vi "results_interface.vi"() -> ()   [LabVIEW 2015]
panel:
  in  "Tab Control":enum32{"Controls", "Insigts", "Debug"}(tab)
  out "Cleaning Up":bool
  out "Calculating Sessions":bool
  out "Total Rate":string
  in  "Velocity Maximum":dbl=100.0 min=0.0 max=100.0
  in  "Experiment ID":string="All"
  in  "Lower Timestamp":timestamp=timestamp(3455817549.4224453 s since 1904-01-01)
  in  "Upper Timestamp":timestamp=timestamp(4308844760.779092 s since 1904-01-01)
  in  "Upper Integer Timestamp":i64=2225999960000 min=1340137854565 max=2040137854565 step=10000000
  in  "Lower Integer Timestamp":i64=1372972749000 min=1340137854565 max=2062085784667 step=10000000
  in  "Dust ID":string="Any"
  in  "Esstimate Dust Quality":cluster{i32, i32}(slide)={2, 5} scale=0.0..5.0
  out "Running":bool
  out "Finished Sessions":bool
  out "Valid Path":bool
  in  "Estimate Session Quality":cluster{i32, i32}(slide)={2, 5} scale=0.0..5.0
  in  "Dust Material":string(combo)="Any Material"
  in  "Velocity Minimun":dbl min=0.0 max=100.0
  in  "Path":path=path "C:/Users/17208/Dust-Accelerator-Database-Analysis/generate_sessions.py"
  in  "End Program":bool
  in  "Calculate Results":bool
  out "?":string="Session Quality Explanation"
  out "?":string="Vecloty Bins Explanation"
  in  "Calculate Results":bool
  in  "Tab Control 2":enum32{"Results Insights", "Results Breakdown"}(tab)
  in  "Tab Control 4":enum32{"Rates", "Particles", "Runtime"}(tab)
  out "results_rates.png":picture
  out "results_particle_count.png":picture
  out "results_runtime.png":picture
  in  "Tab Control 3":T1(tab)
  out "Session Quality Breakdown":picture
  out "Session Particle Quality Breakdown":picture
  out "Session Duration Breakdown":picture
  out "Session Dust Event Count Breakdown":picture
  out "Results Output":string
  out "Request":string
  out "Results Error/Debug":string
  out "Session Generator Output":string
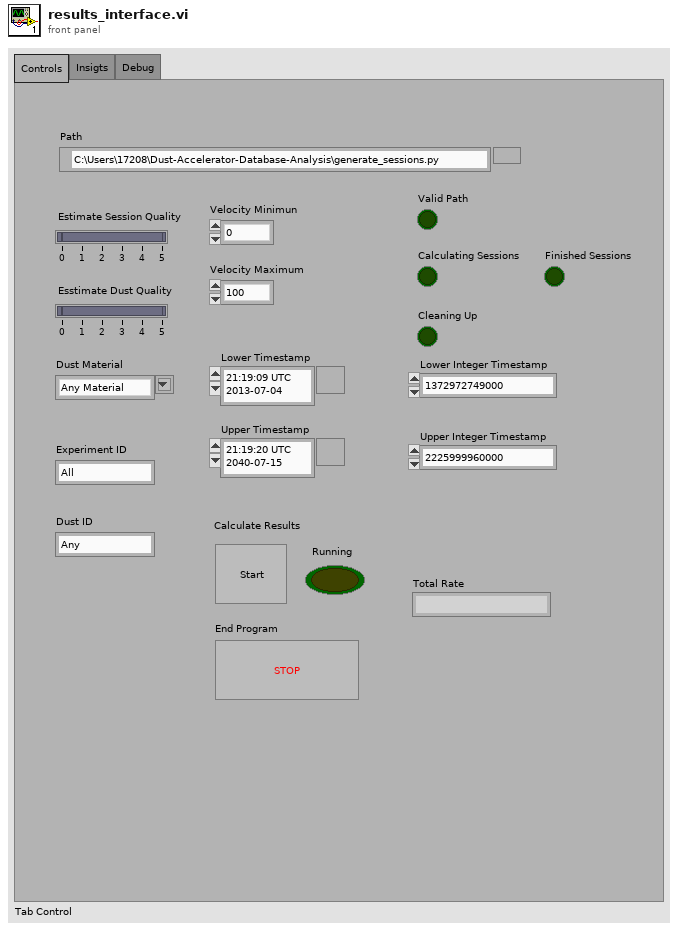
[diagram p1: front panel]
types:
  T1 = enum32{"Session Quality ", "Particle Quality", "Session Duration", "Session Event Counts"}
  T2 = cluster{string, string, string, string, string, string, string}
  T3 = cluster{"Velocity Minimun ":dbl, "Velocity Maximum":dbl}
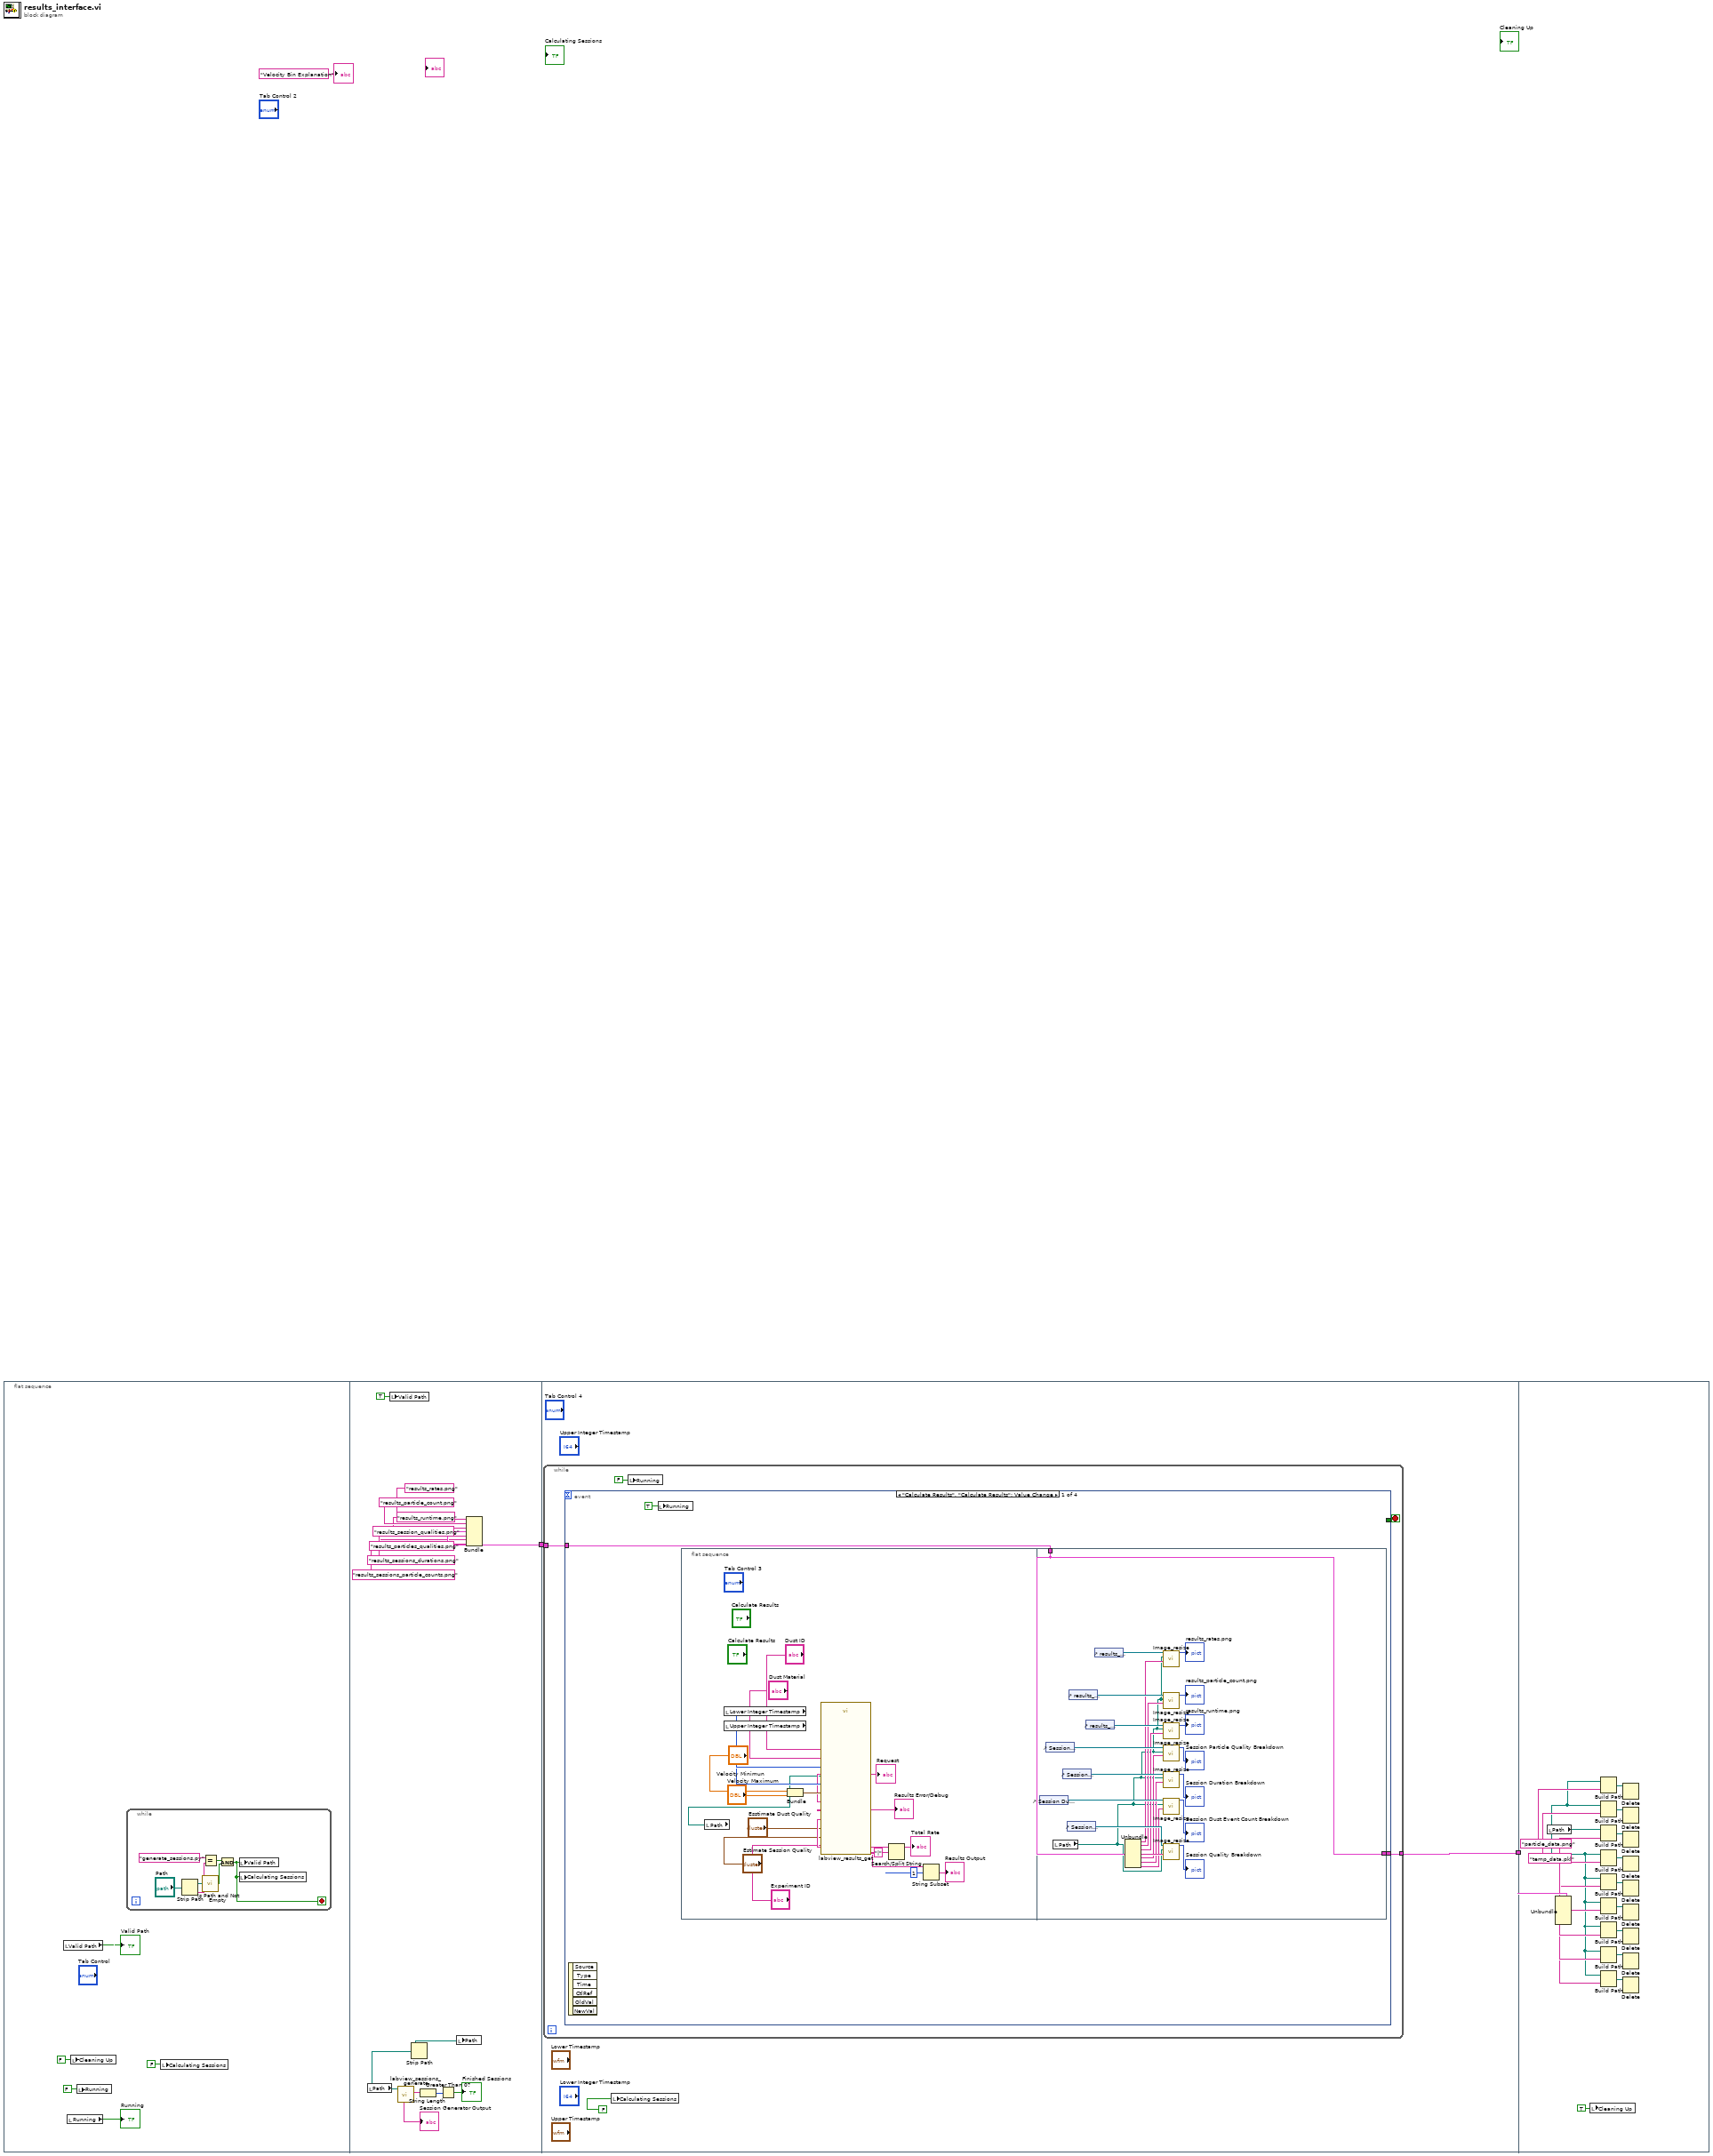
[diagram p0: block diagram]
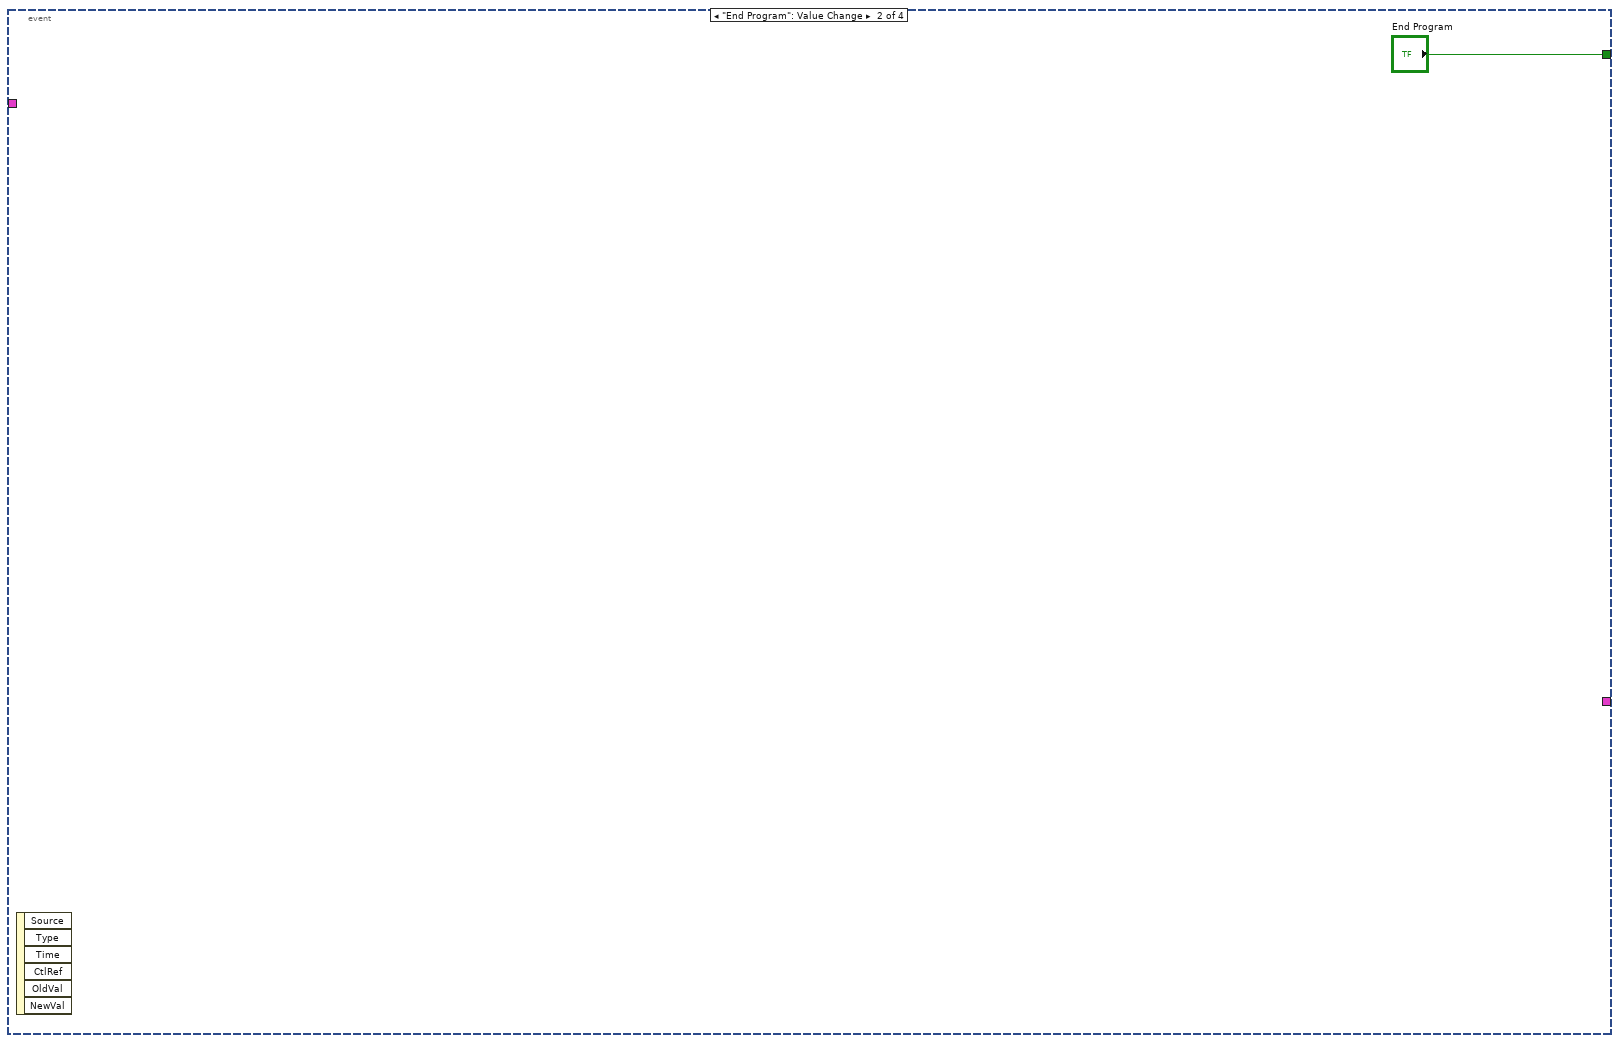
[diagram p2: hidden frame]
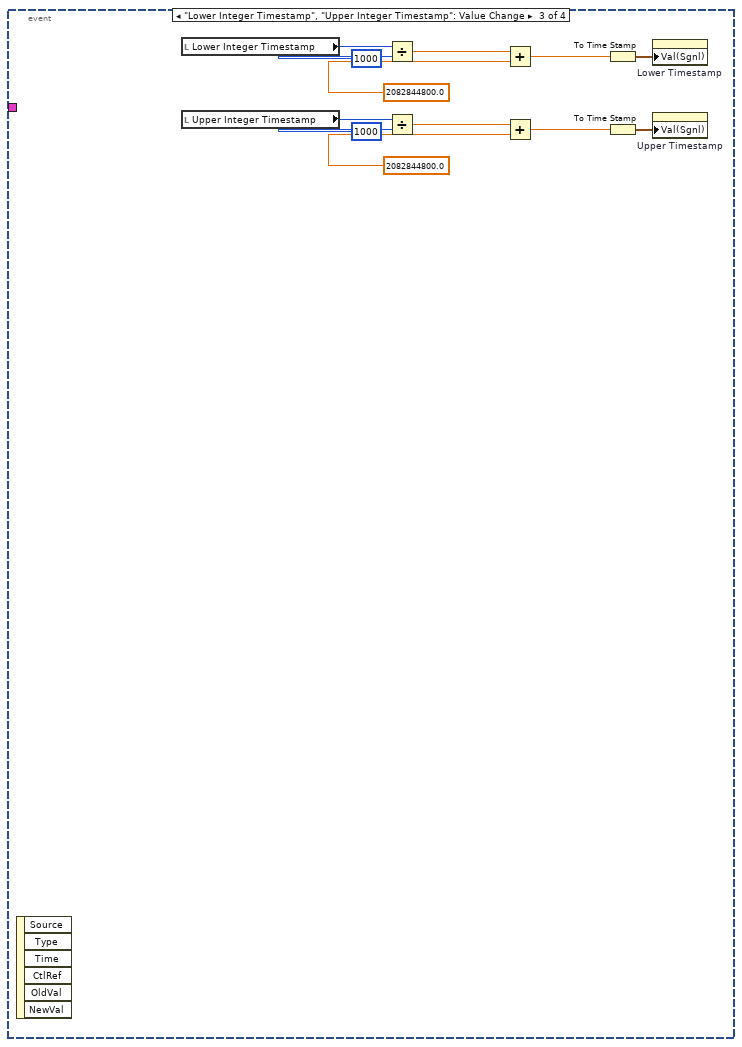
[diagram p3: hidden frame]
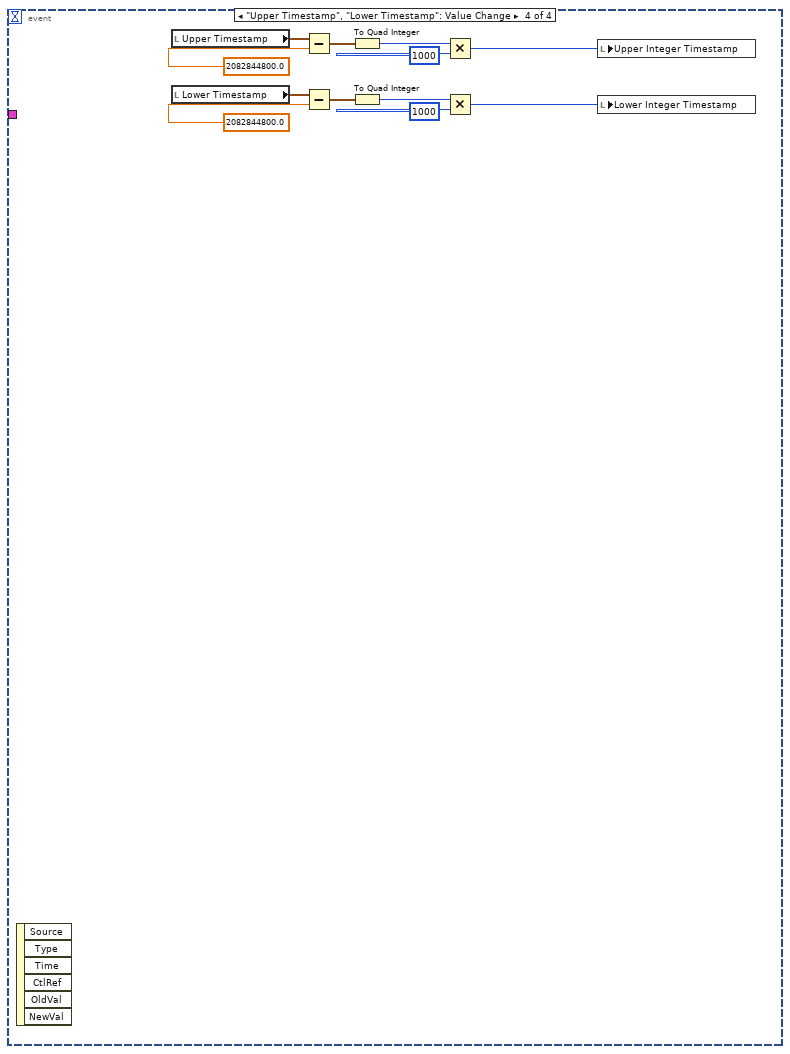
[diagram p4: hidden frame]
diagram:
  n1 = flat-sequence {
    tunnel: [w25] -> w2
    tunnel: w2 -> [w32]
    tunnel: [w31] -> w1
    tunnel: w1 -> [w116]
    frame #0 {
      n2 = local read "Valid Path"() -> (→"Valid Path":bool)
      n3 = local read "Running"() -> (→"Running":bool)
      n4 = local write "Cleaning Up"(FALSE ("Cleaning Up")) -> ()
      n5 = local write "Running"(FALSE) -> ()
      n6 = while {
        stop <- w9 stop-if-true
        n7 = Strip Path(path="Path") -> (stripped path=w10:path, name=w15:string)
        n8 = Equal?(x="generate_sessions.py", y=w15) -> (x = y?=w13:bool)
        n9 = call <vilib>:"Is Path and Not Empty.vi"("path"=w10) -> ("Is Path and Not Empty?"=w12:bool)  [unwired: 4 in]
        n10 = And(x=w13, y=w12) -> (x .and. y?=w9:bool)
        n11 = local write "Valid Path"(w9) -> ()
        n12 = local write "Calculating Sessions"(w9) -> ()
      }
      n13 = local write "Calculating Sessions"(FALSE ("Calculating Sessions")) -> ()
    }
    frame #1 {
      n14 = local read "Path"() -> (w17:path)
      n15 = local write "Valid Path"(TRUE) -> ()
      n16 = call "labview_sessions_generate.vi"("Path"=w17) -> ("Session Generator Output"=w29:string)  [unwired: 10 in]
      "Session Generator Output" <- w29
      n17 = Strip Path(path=w17) -> (stripped path=w16:path)  [unwired: 1 out]
      n18 = String Length(string=w29) -> (length=w28:i32)
      n19 = Greater Than 0?(x=w28) -> (x > 0?=→"Finished Sessions":bool)
      n20 = local write "Path"(w16) -> ()
      n21 = Bundle("results_rates.png", "results_particle_count.png", "results_runtime.png", "results_session_qualities.png", "results_particles_qualities.png", "results_sessions_durations.png", "results_sessions_particle_counts.png") -> (w25:T2)  [unwired: 1 in]
    }
    frame #2 {
      n22 = while {
        tunnel: w32 -> [w35]
        tunnel: [w34] -> w31
        stop <- w33 stop-if-true
        n23 = event shown="[0] \"Calculate Results\", \"Calculate Results\": Value Change" {
          selector: _ -> [_ _ _ _]
          dyn-events: _ -> [_ _ _ _]
          timeout: _ -> [_ _ _ _]
          tunnel: [_ "End Program" _ _] -> w33
          tunnel: w35 -> [w38 _ _ _]
          tunnel: [w37 _ _ _] -> w34
          event "Calculate Results", "Calculate Results": Value Change {
            n24 = event-data() -> ()  [unwired: 1 in, 6 out]
            n25 = local write "Running"(TRUE) -> ()
            n26 = flat-sequence {
              tunnel: w38 -> [w81]
              tunnel: [w81] -> w37
              frame #0 {
                n27 = local read "Path"() -> (w40:path)
                n28 = local read "Lower Integer Timestamp"() -> (w52:i64)
                n29 = local read "Upper Integer Timestamp"() -> (w51:i64)
                n30 = Bundle("Velocity Minimun"="Velocity Minimun", "Velocity Maximum"="Velocity Maximum") -> (w56:T3)  [unwired: 1 in]
                n31 = call "labview_results_get.vi"("Path"=w40, "Dust ID"="Dust ID", "Upper Timestamp"=w51, "Velocity Limits"=w56, "Lower Timestamp"=w52, "Particle Quality"="Esstimate Dust Quality", "Session Quality"="Estimate Session Quality", "Experiment ID"="Experiment ID", "Dust Material"="Dust Material") -> ("Results Output"=w57:string, "Results Error/Debug"=→"Results Error/Debug":string, "Request"=→"Request":string)  [unwired: 16 in]
                n32 = Search/Split String(string=w57, search string/char (-)="|") -> (substring before match=→"Total Rate":string, match + rest of string=w42:string)  [unwired: 1 in, 1 out]
                n33 = String Subset(string=w42, offset (0)=1) -> (substring=→"Results Output":string)  [unwired: 1 in]
              }
              frame #1 {
                n34 = control-ref of="Session Dust Event Count Breakdown"() -> (w67:refnum<vi>)
                n35 = control-ref of="Session Particle Quality Breakdown"() -> (w69:refnum<vi>)
                n36 = local read "Path"() -> (w59:path)
                n37 = control-ref of="Session Duration Breakdown"() -> (w68:refnum<vi>)
                n38 = control-ref of="Session Quality Breakdown"() -> (w70:refnum<vi>)
                n39 = control-ref of="results_particle_count.png"() -> (w72:refnum<vi>)
                n40 = control-ref of="results_runtime.png"() -> (w71:refnum<vi>)
                n41 = control-ref of="results_rates.png"() -> (w73:refnum<vi>)
                n42 = Unbundle(w81) -> (w66:string, w65:string, w64:string, w63:string, w62:string, w61:string, w60:string)
                n43 = call "Image_resize.vi"("String"=w66, "stripped path"=w59, "Picture in"=w73) -> ("2D Picture"=→"results_rates.png":picture)  [unwired: 8 in]
                n44 = call "Image_resize.vi"("String"=w65, "stripped path"=w59, "Picture in"=w72) -> ("2D Picture"=→"results_particle_count.png":picture)  [unwired: 8 in]
                n45 = call "Image_resize.vi"("String"=w64, "stripped path"=w59, "Picture in"=w71) -> ("2D Picture"=→"results_runtime.png":picture)  [unwired: 8 in]
                n46 = call "Image_resize.vi"("String"=w62, "stripped path"=w59, "Picture in"=w69) -> ("2D Picture"=→"Session Particle Quality Breakdown":picture)  [unwired: 8 in]
                n47 = call "Image_resize.vi"("String"=w61, "stripped path"=w59, "Picture in"=w68) -> ("2D Picture"=→"Session Duration Breakdown":picture)  [unwired: 8 in]
                n48 = call "Image_resize.vi"("String"=w60, "stripped path"=w59, "Picture in"=w67) -> ("2D Picture"=→"Session Dust Event Count Breakdown":picture)  [unwired: 8 in]
                n49 = call "Image_resize.vi"("String"=w63, "stripped path"=w59, "Picture in"=w70) -> ("2D Picture"=→"Session Quality Breakdown":picture)  [unwired: 8 in]
              }
            }
          }
          event "End Program": Value Change {
            n50 = event-data() -> ()  [unwired: 1 in, 6 out]
          }
          event "Lower Integer Timestamp", "Upper Integer Timestamp": Value Change {
            n51 = event-data() -> ()  [unwired: 1 in, 6 out]
            n52 = local read "Lower Integer Timestamp"() -> (w93:i64)
            n53 = local read "Upper Integer Timestamp"() -> (w91:i64)
            n54 = Divide(x=w93, y=1000) -> (x/y=w85:dbl)
            n55 = Divide(x=w91, y=1000) -> (x/y=w87:dbl)
            n56 = Add(x=w85, y=2082844800.0) -> (x+y=w83:dbl)
            n57 = Add(x=w87, y=2082844800.0) -> (x+y=w86:dbl)
            n58 = To Time Stamp(1:w83) -> (0:w89:timestamp)
            n59 = To Time Stamp(1:w86) -> (0:w90:timestamp)
            n60 = property on="Lower Timestamp" class="AbsTime (strict)"("Val(Sgnl)"=w89) -> ()  [unwired: 2 in, 2 out]
            n61 = property on="Upper Timestamp" class="AbsTime (strict)"("Val(Sgnl)"=w90) -> ()  [unwired: 2 in, 2 out]
          }
          event "Upper Timestamp", "Lower Timestamp": Value Change {
            n62 = event-data() -> ()  [unwired: 1 in, 6 out]
            n63 = local read "Upper Timestamp"() -> (w95:timestamp)
            n64 = local read "Lower Timestamp"() -> (w96:timestamp)
            n65 = Subtract(x=w95, y=2082844800.0) -> (x-y=w102:timestamp)
            n66 = Subtract(x=w96, y=2082844800.0) -> (x-y=w103:timestamp)
            n67 = To Quad Integer(1:w102) -> (0:w99:i64)
            n68 = To Quad Integer(1:w103) -> (0:w101:i64)
            n69 = Multiply(x=w99, y=1000) -> (x*y=w98:i64)
            n70 = Multiply(x=w101, y=1000) -> (x*y=w100:i64)
            n71 = local write "Upper Integer Timestamp"(w98) -> ()
            n72 = local write "Lower Integer Timestamp"(w100) -> ()
          }
        }
        n73 = local write "Running"(FALSE ("Boolean")) -> ()
      }
      n74 = local write "Calculating Sessions"(FALSE ("Calculating Sessions")) -> ()
    }
    frame #3 {
      n75 = local read "Path"() -> (w107:path)
      n76 = Unbundle(w116) -> (w115:string, w114:string, w113:string, w112:string, w111:string, w110:string, w109:string)
      n77 = local write "Cleaning Up"(TRUE ("Cleaning Up")) -> ()
      n78 = Build Path(base path=w107, name or relative path="particle_data.png") -> (appended path=w125:path)
      n79 = Build Path(base path=w107, name or relative path="temp_data.pkl") -> (appended path=w127:path)
      n80 = Build Path(base path=w107, name or relative path=w115) -> (appended path=w122:path)
      n81 = Build Path(base path=w107, name or relative path=w114) -> (appended path=w121:path)
      n82 = Build Path(base path=w107, name or relative path=w113) -> (appended path=w123:path)
      n83 = Build Path(base path=w107, name or relative path=w112) -> (appended path=w120:path)
      n84 = Build Path(base path=w107, name or relative path=w111) -> (appended path=w119:path)
      n85 = Build Path(base path=w107, name or relative path=w110) -> (appended path=w118:path)
      n86 = Build Path(base path=w107, name or relative path=w109) -> (appended path=w117:path)
      n87 = Delete(path (use dialog)=w125) -> ()  [unwired: 4 in, 3 out]
      n88 = Delete(path (use dialog)=w127) -> ()  [unwired: 4 in, 3 out]
      n89 = Delete(path (use dialog)=w122) -> ()  [unwired: 4 in, 3 out]
      n90 = Delete(path (use dialog)=w121) -> ()  [unwired: 4 in, 3 out]
      n91 = Delete(path (use dialog)=w123) -> ()  [unwired: 4 in, 3 out]
      n92 = Delete(path (use dialog)=w120) -> ()  [unwired: 4 in, 3 out]
      n93 = Delete(path (use dialog)=w119) -> ()  [unwired: 4 in, 3 out]
      n94 = Delete(path (use dialog)=w118) -> ()  [unwired: 4 in, 3 out]
      n95 = Delete(path (use dialog)=w117) -> ()  [unwired: 4 in, 3 out]
    }
  }
  "?" <- "Velocity Bin Explanation"
